vi "WVDIAL_1_AMCS_2.0.vi"() -> ()   [LabVIEW 2012]
uses:
  <vilib>/Analysis/baseanly.llb/Mean (DBL).vi
  NCAR_DIAL_Labview/AMCS_Data.vi
  AmcsUsb.dll
  <vilib>/Analysis/NI_AALBase.lvlib
panel:
  out "x/y":dbl=nan
  out "Narrow Ratio":dbl(graph)=nan
  in  "Near Ch Offline mult":dbl=0.85
  out "size(s)":i32=1121
  in  "Channels":u32=4
  in  "Data Reads":i32=279
  out "Loop Count":i32=835
  in  "TC Start":i32=2 min=1 max=1894
  in  "TC Length":i32=15 min=2 max=280
  out "TC background sub over length":cluster{dbl, dbl, dbl, dbl}(graph)={0.0, 0.0, 2617.010638297873, 3738.4361702127662}
  out "return type":i32
  out "Raw Uncorrected Return":u16[][](graph)=[[0, 0, 0, 0, 0, 0, 0, 0, 0, 0, 0, 0, 0, 0, 0, 0, 0, 0, 0, 0, 0, 0, 0, 0, 0, 0, 0, 0, 0, 0, 0, 0, 0, 0, 0, 0, 0, 0, 0, 0, 0, 0, 0, 0, 0, 0, 0, 0, 0, 0, 0, 0, 0, 0, 0, 0, 0, 0, 0, 0, 0, 0, 0, 0, 0, 0, 0, 0, 0, 0, 0, 0, 0, 0, 0, 0, 0, 0, 0, 0, 0, 0, 0, 0, 0, 0, 0, 0, 0, 0, 0, 0, 0, 0, 0, 0, 0, 0, 0, 0, 0, 0, 0, 0, 0, 0, 0, 0, 0, 0, 0, 0, 0, 0, 0, 0, 0, 0, 0, 0, 0, 0, 0, 0, 0, 0, 0, 0, 0, 0, 0, 0, 0, 0, 0, 0, 0, 0, 0, 0, 0, 0, 0, 0, 0, 0, 0, 0, 0, 0, 0, 0, 0, 0, 0, 0, 0, 0, 0, 0, 0, 0, 0, 0, 0, 0, 0, 0, 0, 0, 0, 0, 0, 0, 0, 0, 0, 0, 0, 0, 0, 0, 0, 0, 0, 0, 0, 0, 0, 0, 0, 0, 0, 0, 0, 0, 0, 0, 0, 0, 0, 0, 0, 0, 0, 0, 0, 0, 0, 0, 0, 0, 0, 0, 0, 0, 0, 0, 0, 0, 0, 0, 0, 0, 0, 0, 0, 0, 0, 0, 0, 0, 0, 0, 0, 0, 0, 0, 0, 0, 0, 0, 0, 0, 0, 0, 0, 0, 0, 0, 0, 0, 0, 0, 0, 0, 0, 0, 0, 0, 0, 0, 0, 0, 0, 0, 0, 0, 0, 0, 0, 0, 0, 0, 0, 0, 0, 0, 0, 0], [0, 0, 0, 0, 0, 0, 0, 0, 0, 0, 0, 0, 0, 0, 0, 0, 0, 0, 0, 0, 0, 0, 0, 0, 0, 0, 0, 0, 0, 0, 0, 0, 0, 0, 0, 0, 0, 0, 0, 0, 0, 0, 0, 0, 0, 0, 0, 0, 0, 0, 0, 0, 0, 0, 0, 0, 0, 0, 0, 0, 0, 0, 0, 0, 0, 0, 0, 0, 0, 0, 0, 0, 0, 0, 0, 0, 0, 0, 0, 0, 0, 0, 0, 0, 0, 0, 0, 0, 0, 0, 0, 0, 0, 0, 0, 0, 0, 0, 0, 0, 0, 0, 0, 0, 0, 0, 0, 0, 0, 0, 0, 0, 0, 0, 0, 0, 0, 0, 0, 0, 0, 0, 0, 0, 0, 0, 0, 0, 0, 0, 0, 0, 0, 0, 0, 0, 0, 0, 0, 0, 0, 0, 0, 0, 0, 0, 0, 0, 0, 0, 0, 0, 0, 0, 0, 0, 0, 0, 0, 0, 0, 0, 0, 0, 0, 0, 0, 0, 0, 0, 0, 0, 0, 0, 0, 0, 0, 0, 0, 0, 0, 0, 0, 0, 0, 0, 0, 0, 0, 0, 0, 0, 0, 0, 0, 0, 0, 0, 0, 0, 0, 0, 0, 0, 0, 0, 0, 0, 0, 0, 0, 0, 0, 0, 0, 0, 0, 0, 0, 0, 0, 0, 0, 0, 0, 0, 0, 0, 0, 0, 0, 0, 0, 0, 0, 0, 0, 0, 0, 0, 0, 0, 0, 0, 0, 0, 0, 0, 0, 0, 0, 0, 0, 0, 0, 0, 0, 0, 0, 0, 0, 0, 0, 0, 0, 0, 0, 0, 0, 0, 0, 0, 0, 0, 0, 0, 0, 0, 0, 0], [16853, 241, 204, 203, 228, 261, 282, 296, 297, 331, 349, 362, 433, 449, 460, 491, 495, 520, 510, 556, 556, 565, 611, 567, 552, 601, 573, 553, 503, 557, 470, 499, 463, 501, 449, 442, 440, 432, 426, 403, 428, 394, 399, 368, 342, 336, 322, 360, 339, 308, 315, 291, 290, 338, 318, 292, 270, 306, 296, 359, 323, 305, 218, 355, 329, 334, 295, 287, 310, 245, 230, 237, 224, 206, 277, 204, 214, 197, 167, 177, 176, 175, 173, 184, 163, 164, 174, 180, 196, 147, 167, 181, 193, 208, 206, 150, 185, 167, 150, 178, 172, 182, 165, 183, 161, 162, 174, 181, 200, 180, 169, 177, 162, 179, 185, 172, 169, 159, 172, 166, 170, 174, 163, 163, 160, 163, 189, 204, 160, 174, 158, 157, 164, 169, 180, 179, 151, 173, 160, 154, 168, 155, 177, 162, 188, 163, 177, 169, 196, 168, 156, 176, 160, 172, 156, 163, 192, 167, 173, 167, 184, 205, 179, 157, 166, 164, 152, 142, 156, 160, 167, 158, 166, 195, 171, 167, 174, 167, 185, 185, 176, 156, 172, 160, 170, 182, 183, 173, 175, 166, 192, 154, 173, 187, 154, 159, 172, 154, 159, 155, 171, 146, 162, 146, 172, 168, 179, 191, 178, 155, 160, 167, 168, 173, 165, 171, 160, 140, 199, 162, 161, 156, 176, 173, 175, 157, 167, 186, 155, 181, 171, 170, 177, 158, 194, 187, 140, 187, 150, 165, 176, 174, 178, 160, 146, 175, 149, 161, 139, 151, 168, 178, 158, 152, 185, 158, 168, 167, 190, 178, 182, 163, 189, 160, 163, 151, 186, 157, 162, 190, 168, 159, 192, 172, 163, 171, 189, 173, 158, 183], [38037, 236, 178, 171, 179, 186, 201, 209, 261, 328, 315, 386, 406, 494, 521, 567, 610, 682, 689, 654, 690, 641, 695, 703, 756, 778, 687, 701, 681, 649, 640, 585, 602, 541, 571, 498, 518, 534, 470, 446, 415, 431, 423, 351, 381, 363, 349, 345, 357, 315, 283, 311, 319, 299, 301, 253, 310, 1200, 3260, 6470, 6733, 4551, 2689, 5021, 10754, 11587, 7963, 7107, 7726, 6654, 4433, 3014, 2917, 2990, 4569, 4723, 2702, 1231, 763, 240, 130, 110, 115, 114, 97, 95, 107, 128, 212, 314, 405, 559, 837, 1180, 1188, 1033, 601, 324, 303, 501, 516, 299, 202, 141, 158, 302, 512, 633, 776, 696, 430, 239, 131, 101, 90, 80, 98, 89, 77, 76, 75, 93, 80, 95, 88, 106, 82, 99, 90, 86, 100, 87, 83, 76, 96, 87, 95, 118, 89, 77, 96, 86, 89, 92, 80, 94, 77, 91, 83, 93, 96, 85, 80, 79, 87, 91, 107, 79, 77, 84, 84, 85, 86, 84, 90, 98, 86, 97, 82, 84, 82, 73, 93, 82, 79, 79, 86, 92, 96, 97, 92, 88, 90, 76, 98, 87, 79, 79, 79, 88, 66, 93, 94, 79, 80, 83, 83, 78, 78, 75, 102, 92, 86, 89, 61, 83, 92, 87, 90, 70, 76, 78, 104, 74, 86, 86, 92, 74, 104, 103, 59, 72, 97, 86, 86, 90, 75, 93, 70, 101, 57, 89, 97, 80, 84, 89, 84, 80, 95, 90, 87, 79, 87, 82, 91, 82, 83, 79, 81, 92, 80, 81, 87, 92, 92, 82, 89, 82, 93, 79, 89, 90, 83, 87, 80, 84, 80, 116, 87, 93, 86, 79, 79, 106, 86, 90, 85, 79, 74, 91]]
  in  "stop":bool
  out "Corrected Return":dbl[][](graph)=[[0.0, 0.0, 0.0, 0.0, 0.0, 0.0, 0.0, 0.0, 0.0, 0.0, 0.0, 0.0, 0.0, 0.0, 0.0, 0.0, 0.0, 0.0, 0.0, 0.0, 0.0, 0.0, 0.0, 0.0, 0.0, 0.0, 0.0, 0.0, 0.0, 0.0, 0.0, 0.0, 0.0, 0.0, 0.0, 0.0, 0.0, 0.0, 0.0, 0.0, 0.0, 0.0, 0.0, 0.0, 0.0, 0.0, 0.0, 0.0, 0.0, 0.0, 0.0, 0.0, 0.0, 0.0, 0.0, 0.0, 0.0, 0.0, 0.0, 0.0, 0.0, 0.0, 0.0, 0.0, 0.0, 0.0, 0.0, 0.0, 0.0, 0.0, 0.0, 0.0, 0.0, 0.0, 0.0, 0.0, 0.0, 0.0, 0.0, 0.0, 0.0, 0.0, 0.0, 0.0, 0.0, 0.0, 0.0, 0.0, 0.0, 0.0, 0.0, 0.0, 0.0, 0.0, 0.0, 0.0, 0.0, 0.0, 0.0, 0.0, 0.0, 0.0, 0.0, 0.0, 0.0, 0.0, 0.0, 0.0, 0.0, 0.0, 0.0, 0.0, 0.0, 0.0, 0.0, 0.0, 0.0, 0.0, 0.0, 0.0, 0.0, 0.0, 0.0, 0.0, 0.0, 0.0, 0.0, 0.0, 0.0, 0.0, 0.0, 0.0, 0.0, 0.0, 0.0, 0.0, 0.0, 0.0, 0.0, 0.0, 0.0, 0.0, 0.0, 0.0, 0.0, 0.0, 0.0, 0.0, 0.0, 0.0, 0.0, 0.0, 0.0, 0.0, 0.0, 0.0, 0.0, 0.0, 0.0, 0.0, 0.0, 0.0, 0.0, 0.0, 0.0, 0.0, 0.0, 0.0, 0.0, 0.0, 0.0, 0.0, 0.0, 0.0, 0.0, 0.0, 0.0, 0.0, 0.0, 0.0, 0.0, 0.0, 0.0, 0.0, 0.0, 0.0, 0.0, 0.0, 0.0, 0.0, 0.0, 0.0, 0.0, 0.0, 0.0, 0.0, 0.0, 0.0, 0.0, 0.0, 0.0, 0.0, 0.0, 0.0, 0.0, 0.0, 0.0, 0.0, 0.0, 0.0, 0.0, 0.0, 0.0, 0.0, 0.0, 0.0, 0.0, 0.0, 0.0, 0.0, 0.0, 0.0, 0.0, 0.0, 0.0, 0.0, 0.0, 0.0, 0.0, 0.0, 0.0, 0.0, 0.0, 0.0, 0.0, 0.0, 0.0, 0.0, 0.0, 0.0, 0.0, 0.0, 0.0, 0.0, 0.0, 0.0, 0.0, 0.0, 0.0, 0.0, 0.0, 0.0, 0.0, 0.0, 0.0, 0.0, 0.0, 0.0, 0.0, 0.0, 0.0, 0.0, 0.0, 0.0, 0.0, 0.0, 0.0, 0.0, 0.0, 0.0, 0.0, 0.0, 0.0, 0.0, 0.0, 0.0, 0.0, 0.0, 0.0, 0.0], [0.0, 0.0, 0.0, 0.0, 0.0, 0.0, 0.0, 0.0, 0.0, 0.0, 0.0, 0.0, 0.0, 0.0, 0.0, 0.0, 0.0, 0.0, 0.0, 0.0, 0.0, 0.0, 0.0, 0.0, 0.0, 0.0, 0.0, 0.0, 0.0, 0.0, 0.0, 0.0, 0.0, 0.0, 0.0, 0.0, 0.0, 0.0, 0.0, 0.0, 0.0, 0.0, 0.0, 0.0, 0.0, 0.0, 0.0, 0.0, 0.0, 0.0, 0.0, 0.0, 0.0, 0.0, 0.0, 0.0, 0.0, 0.0, 0.0, 0.0, 0.0, 0.0, 0.0, 0.0, 0.0, 0.0, 0.0, 0.0, 0.0, 0.0, 0.0, 0.0, 0.0, 0.0, 0.0, 0.0, 0.0, 0.0, 0.0, 0.0, 0.0, 0.0, 0.0, 0.0, 0.0, 0.0, 0.0, 0.0, 0.0, 0.0, 0.0, 0.0, 0.0, 0.0, 0.0, 0.0, 0.0, 0.0, 0.0, 0.0, 0.0, 0.0, 0.0, 0.0, 0.0, 0.0, 0.0, 0.0, 0.0, 0.0, 0.0, 0.0, 0.0, 0.0, 0.0, 0.0, 0.0, 0.0, 0.0, 0.0, 0.0, 0.0, 0.0, 0.0, 0.0, 0.0, 0.0, 0.0, 0.0, 0.0, 0.0, 0.0, 0.0, 0.0, 0.0, 0.0, 0.0, 0.0, 0.0, 0.0, 0.0, 0.0, 0.0, 0.0, 0.0, 0.0, 0.0, 0.0, 0.0, 0.0, 0.0, 0.0, 0.0, 0.0, 0.0, 0.0, 0.0, 0.0, 0.0, 0.0, 0.0, 0.0, 0.0, 0.0, 0.0, 0.0, 0.0, 0.0, 0.0, 0.0, 0.0, 0.0, 0.0, 0.0, 0.0, 0.0, 0.0, 0.0, 0.0, 0.0, 0.0, 0.0, 0.0, 0.0, 0.0, 0.0, 0.0, 0.0, 0.0, 0.0, 0.0, 0.0, 0.0, 0.0, 0.0, 0.0, 0.0, 0.0, 0.0, 0.0, 0.0, 0.0, 0.0, 0.0, 0.0, 0.0, 0.0, 0.0, 0.0, 0.0, 0.0, 0.0, 0.0, 0.0, 0.0, 0.0, 0.0, 0.0, 0.0, 0.0, 0.0, 0.0, 0.0, 0.0, 0.0, 0.0, 0.0, 0.0, 0.0, 0.0, 0.0, 0.0, 0.0, 0.0, 0.0, 0.0, 0.0, 0.0, 0.0, 0.0, 0.0, 0.0, 0.0, 0.0, 0.0, 0.0, 0.0, 0.0, 0.0, 0.0, 0.0, 0.0, 0.0, 0.0, 0.0, 0.0, 0.0, 0.0, 0.0, 0.0, 0.0, 0.0, 0.0, 0.0, 0.0, 0.0, 0.0, 0.0, 0.0, 0.0, 0.0, 0.0, 0.0, 0.0, 0.0, 0.0, 0.0, 0.0, 0.0, 0.0], [16684.73404255319, 72.7340425531915, 35.7340425531915, 34.7340425531915, 59.7340425531915, 92.7340425531915, 113.7340425531915, 127.7340425531915, 128.7340425531915, 162.7340425531915, 180.7340425531915, 193.7340425531915, 264.7340425531915, 280.7340425531915, 291.7340425531915, 322.7340425531915, 326.7340425531915, 351.7340425531915, 341.7340425531915, 387.7340425531915, 387.7340425531915, 396.7340425531915, 442.7340425531915, 398.7340425531915, 383.7340425531915, 432.7340425531915, 404.7340425531915, 384.7340425531915, 334.7340425531915, 388.7340425531915, 301.7340425531915, 330.7340425531915, 294.7340425531915, 332.7340425531915, 280.7340425531915, 273.7340425531915, 271.7340425531915, 263.7340425531915, 257.7340425531915, 234.7340425531915, 259.7340425531915, 225.7340425531915, 230.7340425531915, 199.7340425531915, 173.7340425531915, 167.7340425531915, 153.7340425531915, 191.7340425531915, 170.7340425531915, 139.7340425531915, 146.7340425531915, 122.7340425531915, 121.7340425531915, 169.7340425531915, 149.7340425531915, 123.7340425531915, 101.7340425531915, 137.7340425531915, 127.7340425531915, 190.7340425531915, 154.7340425531915, 136.7340425531915, 49.7340425531915, 186.7340425531915, 160.7340425531915, 165.7340425531915, 126.7340425531915, 118.7340425531915, 141.7340425531915, 76.7340425531915, 61.7340425531915, 68.7340425531915, 55.7340425531915, 37.7340425531915, 108.7340425531915, 35.7340425531915, 45.7340425531915, 28.7340425531915, -1.2659574468084998, 8.7340425531915, 7.7340425531915, 6.7340425531915, 4.7340425531915, 15.7340425531915, -5.2659574468085, -4.2659574468085, 5.7340425531915, 11.7340425531915, 27.7340425531915, -21.2659574468085, -1.2659574468084998, 12.7340425531915, 24.7340425531915, 39.7340425531915, 37.7340425531915, -18.2659574468085, 16.7340425531915, -1.2659574468084998, -18.2659574468085, 9.7340425531915, 3.7340425531915002, 13.7340425531915, -3.2659574468084998, 14.7340425531915, -7.2659574468085, -6.2659574468085, 5.7340425531915, 12.7340425531915, 31.7340425531915, 11.7340425531915, 0.7340425531915002, 8.7340425531915, -6.2659574468085, 10.7340425531915, 16.7340425531915, 3.7340425531915002, 0.7340425531915002, -9.2659574468085, 3.7340425531915002, -2.2659574468084998, 1.7340425531915002, 5.7340425531915, -5.2659574468085, -5.2659574468085, -8.2659574468085, -5.2659574468085, 20.7340425531915, 35.7340425531915, -8.2659574468085, 5.7340425531915, -10.2659574468085, -11.2659574468085, -4.2659574468085, 0.7340425531915002, 11.7340425531915, 10.7340425531915, -17.2659574468085, 4.7340425531915, -8.2659574468085, -14.2659574468085, -0.26595744680849975, -13.2659574468085, 8.7340425531915, -6.2659574468085, 19.7340425531915, -5.2659574468085, 8.7340425531915, 0.7340425531915002, 27.7340425531915, -0.26595744680849975, -12.2659574468085, 7.7340425531915, -8.2659574468085, 3.7340425531915002, -12.2659574468085, -5.2659574468085, 23.7340425531915, -1.2659574468084998, 4.7340425531915, -1.2659574468084998, 15.7340425531915, 36.7340425531915, 10.7340425531915, -11.2659574468085, -2.2659574468084998, -4.2659574468085, -16.2659574468085, -26.2659574468085, -12.2659574468085, -8.2659574468085, -1.2659574468084998, -10.2659574468085, -2.2659574468084998, 26.7340425531915, 2.7340425531915002, -1.2659574468084998, 5.7340425531915, -1.2659574468084998, 16.7340425531915, 16.7340425531915, 7.7340425531915, -12.2659574468085, 3.7340425531915002, -8.2659574468085, 1.7340425531915002, 13.7340425531915, 14.7340425531915, 4.7340425531915, 6.7340425531915, -2.2659574468084998, 23.7340425531915, -14.2659574468085, 4.7340425531915, 18.7340425531915, -14.2659574468085, -9.2659574468085, 3.7340425531915002, -14.2659574468085, -9.2659574468085, -13.2659574468085, 2.7340425531915002, -22.2659574468085, -6.2659574468085, -22.2659574468085, 3.7340425531915002, -0.26595744680849975, 10.7340425531915, 22.7340425531915, 9.7340425531915, -13.2659574468085, -8.2659574468085, -1.2659574468084998, -0.26595744680849975, 4.7340425531915, -3.2659574468084998, 2.7340425531915002, -8.2659574468085, -28.2659574468085, 30.7340425531915, -6.2659574468085, -7.2659574468085, -12.2659574468085, 7.7340425531915, 4.7340425531915, 6.7340425531915, -11.2659574468085, -1.2659574468084998, 17.7340425531915, -13.2659574468085, 12.7340425531915, 2.7340425531915002, 1.7340425531915002, 8.7340425531915, -10.2659574468085, 25.7340425531915, 18.7340425531915, -28.2659574468085, 18.7340425531915, -18.2659574468085, -3.2659574468084998, 7.7340425531915, 5.7340425531915, 9.7340425531915, -8.2659574468085, -22.2659574468085, 6.7340425531915, -19.2659574468085, -7.2659574468085, -29.2659574468085, -17.2659574468085, -0.26595744680849975, 9.7340425531915, -10.2659574468085, -16.2659574468085, 16.7340425531915, -10.2659574468085, -0.26595744680849975, -1.2659574468084998, 21.7340425531915, 9.7340425531915, 13.7340425531915, -5.2659574468085, 20.7340425531915, -8.2659574468085, -5.2659574468085, -17.2659574468085, 17.7340425531915, -11.2659574468085, -6.2659574468085, 21.7340425531915, -0.26595744680849975, -9.2659574468085, 23.7340425531915, 3.7340425531915002, -5.2659574468085, 2.7340425531915002, 20.7340425531915, 4.7340425531915, -10.2659574468085, 14.7340425531915], [32259.281382978723, 128.4313829787234, 79.13138297872341, 73.1813829787234, 79.9813829787234, 85.9313829787234, 98.6813829787234, 105.4813829787234, 149.6813829787234, 206.6313829787234, 195.58138297872338, 255.93138297872338, 272.9313829787234, 347.7313829787234, 370.6813829787234, 409.7813829787234, 446.3313829787234, 507.53138297872346, 513.4813829787234, 483.73138297872345, 514.3313829787235, 472.68138297872343, 518.5813829787235, 525.3813829787234, 570.4313829787234, 589.1313829787234, 511.78138297872346, 523.6813829787234, 506.68138297872343, 479.48138297872345, 471.8313829787234, 425.0813829787234, 439.53138297872346, 387.6813829787234, 413.1813829787234, 351.13138297872337, 368.13138297872337, 381.7313829787234, 327.3313829787234, 306.9313829787234, 280.5813829787234, 294.1813829787234, 287.38138297872337, 226.18138297872338, 251.68138297872338, 236.3813829787234, 224.4813829787234, 221.08138297872338, 231.2813829787234, 195.58138297872338, 168.3813829787234, 192.1813829787234, 198.9813829787234, 181.9813829787234, 183.6813829787234, 142.8813829787234, 191.33138297872338, 947.8313829787235, 2698.8313829787235, 5427.331382978723, 5650.881382978723, 3796.181382978723, 2213.4813829787236, 4195.681382978723, 9068.731382978724, 9776.781382978723, 6696.381382978723, 5968.781382978723, 6494.9313829787225, 5583.731382978723, 3695.8813829787227, 2489.7313829787236, 2407.2813829787233, 2469.3313829787235, 3811.481382978723, 3942.3813829787227, 2224.5313829787233, 974.1813829787234, 576.3813829787234, 131.83138297872338, 38.33138297872341, 21.331382978723408, 25.581382978723408, 24.73138297872341, 10.281382978723409, 8.58138297872341, 18.781382978723407, 36.63138297872341, 108.0313829787234, 194.7313829787234, 272.0813829787234, 402.9813829787234, 639.2813829787234, 930.8313829787235, 937.6313829787234, 805.8813829787234, 438.68138297872343, 203.2313829787234, 185.3813829787234, 353.6813829787234, 366.4313829787234, 181.9813829787234, 99.5313829787234, 47.681382978723406, 62.13138297872341, 184.5313829787234, 363.0313829787234, 465.8813829787234, 587.4313829787234, 519.4313829787234, 293.3313829787234, 130.9813829787234, 39.181382978723406, 13.68138297872341, 4.331382978723409, -4.1686170212765905, 11.131382978723408, 3.481382978723409, -6.71861702127659, -7.568617021276591, -8.41861702127659, 6.881382978723409, -4.1686170212765905, 8.58138297872341, 2.631382978723409, 17.93138297872341, -2.4686170212765908, 11.981382978723408, 4.331382978723409, 0.9313829787234091, 12.83138297872341, 1.781382978723409, -1.618617021276591, -7.568617021276591, 9.43138297872341, 1.781382978723409, 8.58138297872341, 28.13138297872341, 3.481382978723409, -6.71861702127659, 9.43138297872341, 0.9313829787234091, 3.481382978723409, 6.031382978723409, -4.1686170212765905, 7.731382978723409, -6.71861702127659, 5.181382978723409, -1.618617021276591, 6.881382978723409, 9.43138297872341, 0.08138297872340913, -4.1686170212765905, -5.018617021276591, 1.781382978723409, 5.181382978723409, 18.781382978723407, -5.018617021276591, -6.71861702127659, -0.7686170212765908, -0.7686170212765908, 0.08138297872340913, 0.9313829787234091, -0.7686170212765908, 4.331382978723409, 11.131382978723408, 0.9313829787234091, 10.281382978723409, -2.4686170212765908, -0.7686170212765908, -2.4686170212765908, -10.11861702127659, 6.881382978723409, -2.4686170212765908, -5.018617021276591, -5.018617021276591, 0.9313829787234091, 6.031382978723409, 9.43138297872341, 10.281382978723409, 6.031382978723409, 2.631382978723409, 4.331382978723409, -7.568617021276591, 11.131382978723408, 1.781382978723409, -5.018617021276591, -5.018617021276591, -5.018617021276591, 2.631382978723409, -16.06861702127659, 6.881382978723409, 7.731382978723409, -5.018617021276591, -4.1686170212765905, -1.618617021276591, -1.618617021276591, -5.868617021276591, -5.868617021276591, -8.41861702127659, 14.531382978723409, 6.031382978723409, 0.9313829787234091, 3.481382978723409, -20.31861702127659, -1.618617021276591, 6.031382978723409, 1.781382978723409, 4.331382978723409, -12.66861702127659, -7.568617021276591, -5.868617021276591, 16.23138297872341, -9.26861702127659, 0.9313829787234091, 0.9313829787234091, 6.031382978723409, -9.26861702127659, 16.23138297872341, 15.381382978723408, -22.01861702127659, -10.968617021276591, 10.281382978723409, 0.9313829787234091, 0.9313829787234091, 4.331382978723409, -8.41861702127659, 6.881382978723409, -12.66861702127659, 13.68138297872341, -23.71861702127659, 3.481382978723409, 10.281382978723409, -4.1686170212765905, -0.7686170212765908, 3.481382978723409, -0.7686170212765908, -4.1686170212765905, 8.58138297872341, 4.331382978723409, 1.781382978723409, -5.018617021276591, 1.781382978723409, -2.4686170212765908, 5.181382978723409, -2.4686170212765908, -1.618617021276591, -5.018617021276591, -3.318617021276591, 6.031382978723409, -4.1686170212765905, -3.318617021276591, 1.781382978723409, 6.031382978723409, 6.031382978723409, -2.4686170212765908, 3.481382978723409, -2.4686170212765908, 6.881382978723409, -5.018617021276591, 3.481382978723409, 4.331382978723409, -1.618617021276591, 1.781382978723409, -4.1686170212765905, -0.7686170212765908, -4.1686170212765905, 26.43138297872341, 1.781382978723409, 6.881382978723409, 0.9313829787234091, -5.018617021276591, -5.018617021276591, 17.93138297872341, 0.9313829787234091, 4.331382978723409, 0.08138297872340913, -5.018617021276591, -9.26861702127659, 5.181382978723409]] caption="Corrected Signal"
  out "Max. Rep. Rate (Hz)":dbl=7091.695624423801
  out "Data Collection Time per Column":dbl=2.00004285
  out "Minimum Sync Pulse Period(µs)":dbl=141.01 format="%.2f"
  in  "y units":u16(ring) items=["Bin #", "Sampling Time(µs)", "Range(m)"]
  in  "Time Resolution Per Bin(ns)":u16=500 min=5 max=1063 step=1
  in  "Number of Accumulates":u32=14285 min=1 max=32767 step=1
  in  "Pulse A Polarity":enum16{"Low", "High"}(ring)=enum."High"
  in  "Sync Pulse Polarity":enum32{"Low", "High"}(ring)=enum."High"
  in  "Accumulation Delay(ns)":u16=10 min=10 max=1270 step=1
  in  "Pulse B Delay(ns)":u32=170000 min=80 max=327600 step=1
  in  "Pulse A Delay(ns)":u32=1040 min=80 max=327600
  in  "bins":u32=280 min=2 max=4095 step=1
  out "y offset":u16=10
  in  "ns scale":u16=500
  in  "Pulse B Polarity":enum16{"Low", "High"}(ring)=enum."High"
  out "Running?":bool
  out "Device ID":u32
  out "Open?":bool=TRUE
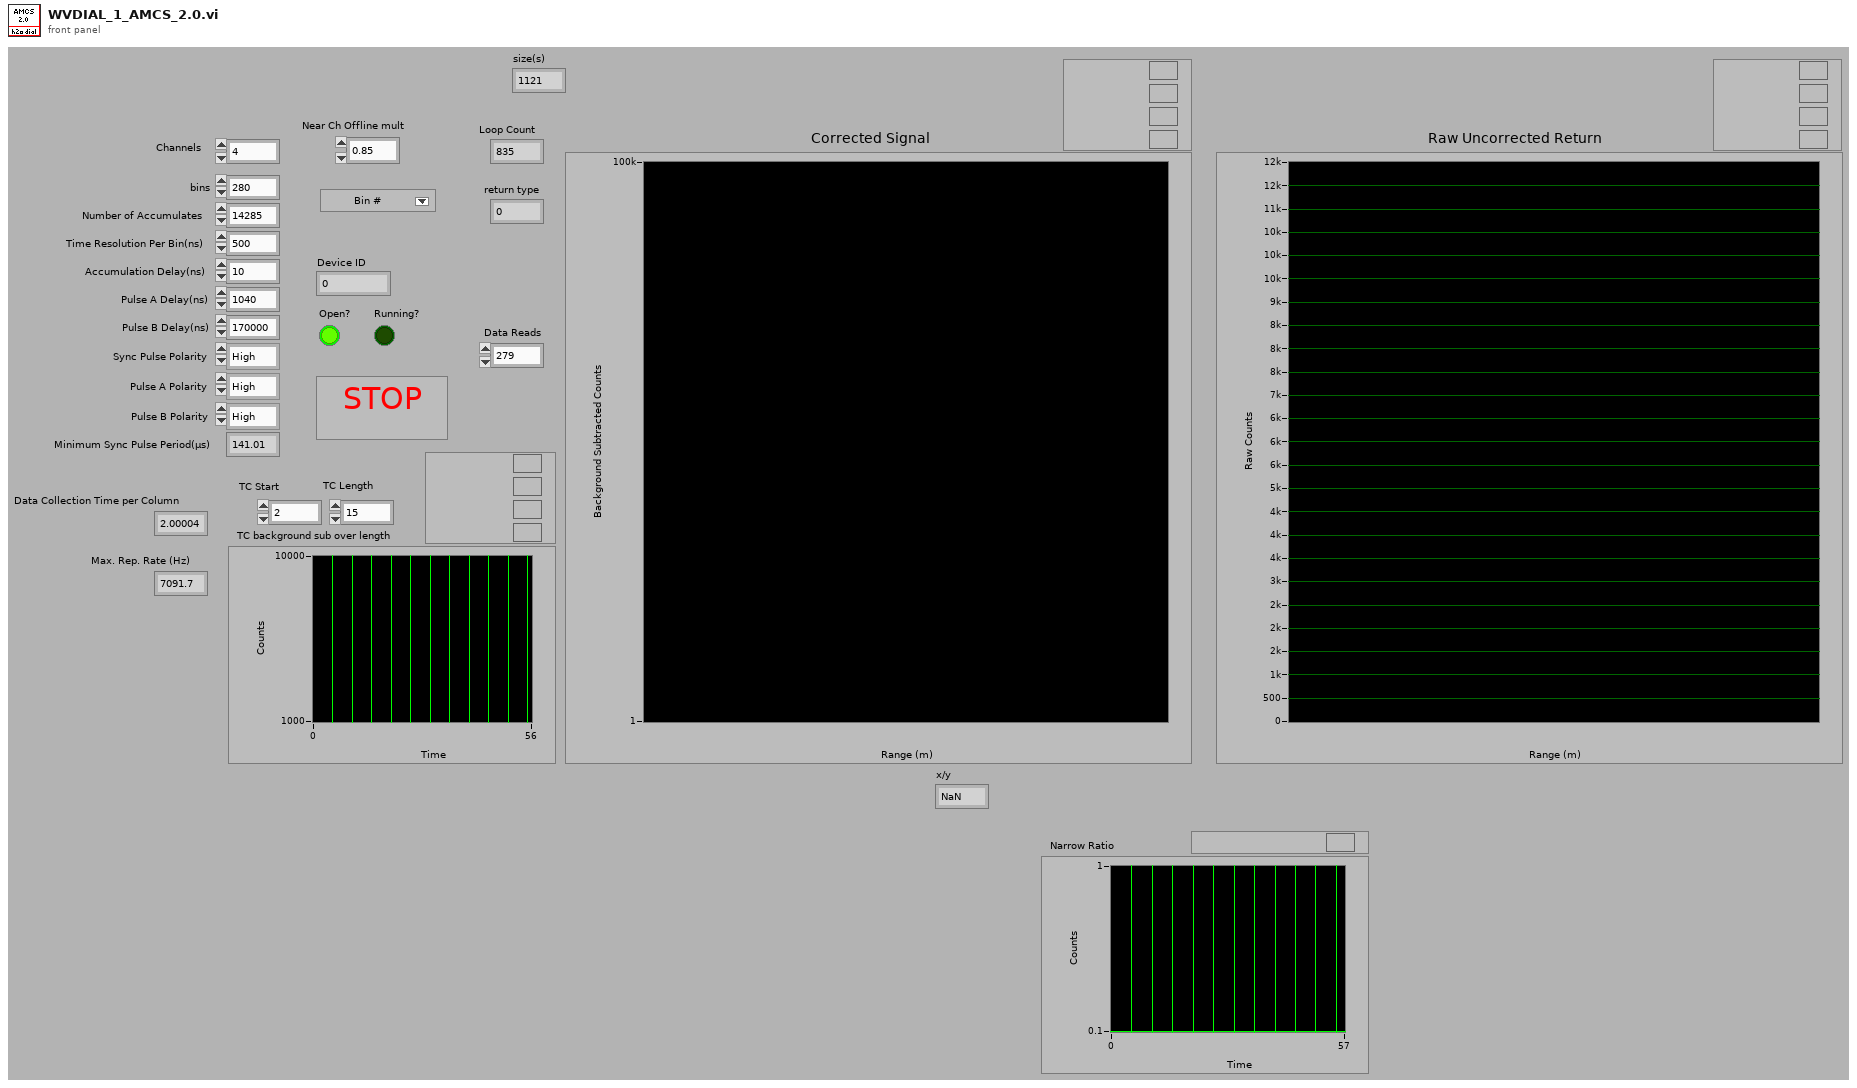
[diagram p1: front panel]
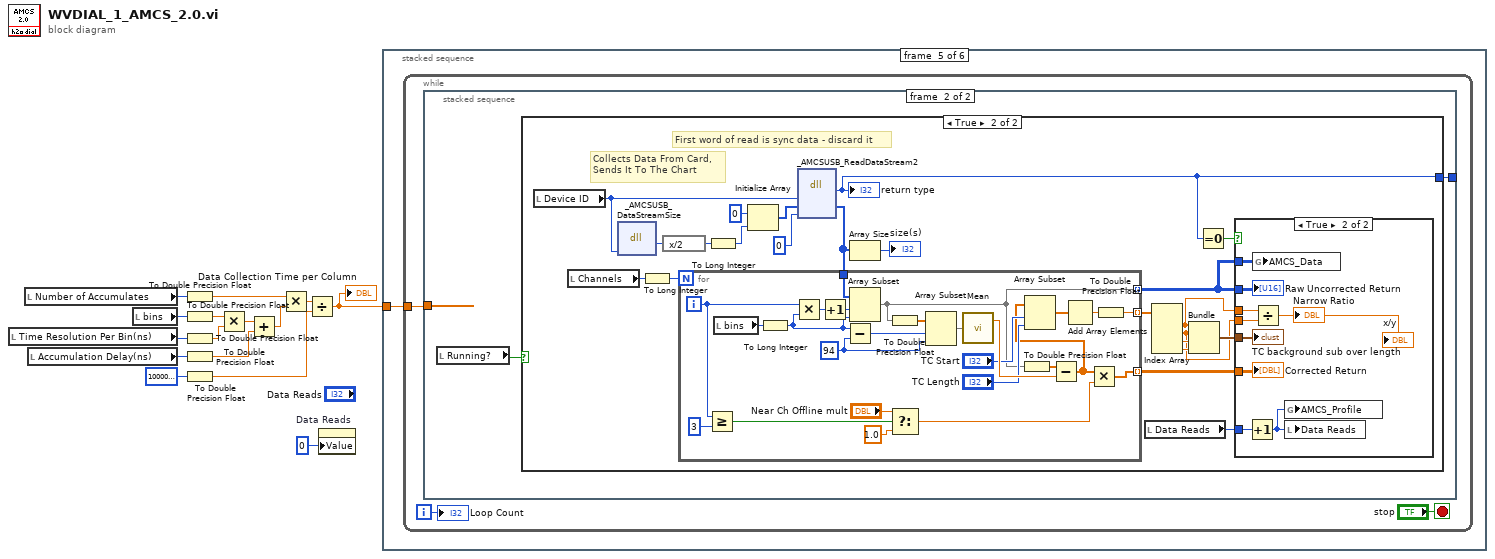
[diagram p0: block diagram]
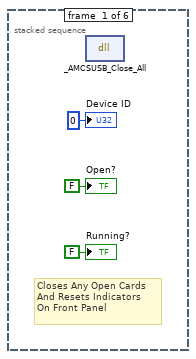
[diagram p2: hidden frame]
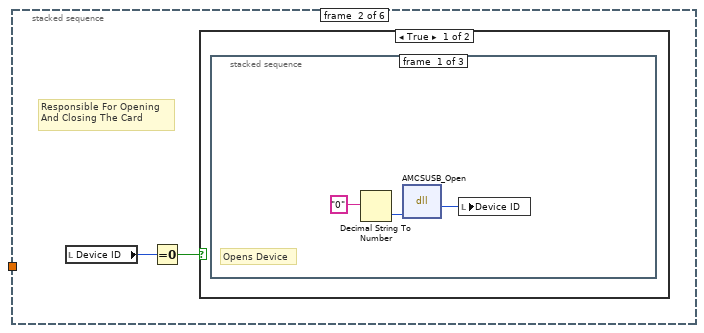
[diagram p3: hidden frame]
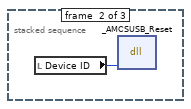
[diagram p4: hidden frame]
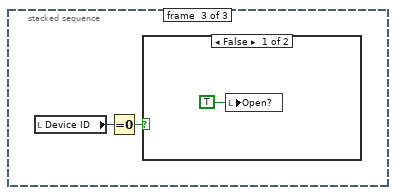
[diagram p5: hidden frame]
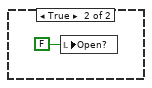
[diagram p6: hidden frame]
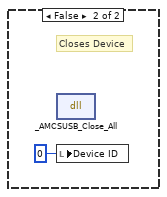
[diagram p7: hidden frame]
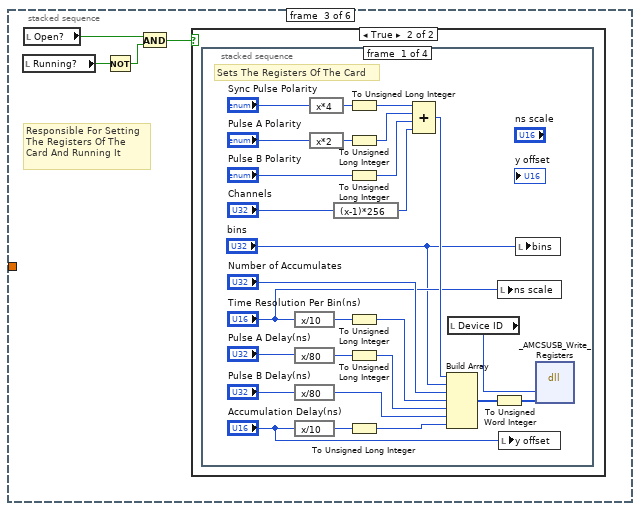
[diagram p8: hidden frame]
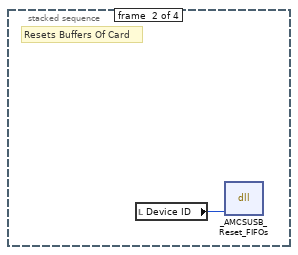
[diagram p10: hidden frame]
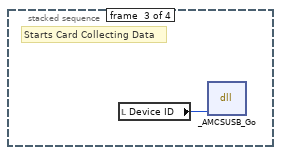
[diagram p11: hidden frame]
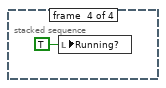
[diagram p12: hidden frame]
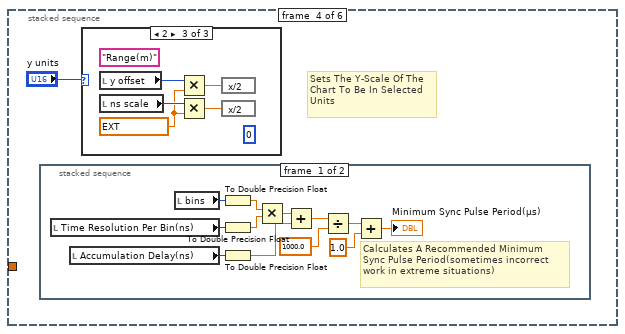
[diagram p13: hidden frame]
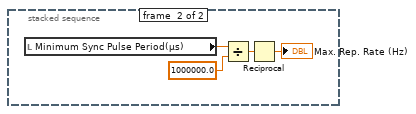
[diagram p14: hidden frame]
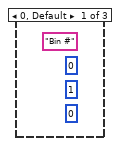
[diagram p15: hidden frame]
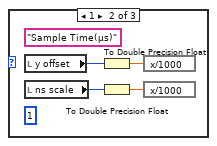
[diagram p16: hidden frame]
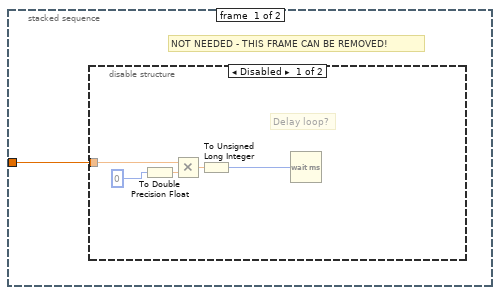
[diagram p17: hidden frame]
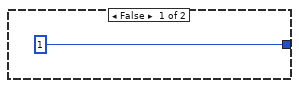
[diagram p19: hidden frame]
diagram:
  n1 = local read "Time Resolution Per Bin(ns)"() -> (w4:u16)
  n2 = local read "Number of Accumulates"() -> (w11:u32)
  n3 = local read "Accumulation Delay(ns)"() -> (w2:u16)
  n4 = local read "bins"() -> (w6:u32)
  n5 = To Double Precision Float(number=w11) -> (double precision float=w10:dbl)
  n6 = To Double Precision Float(number=w6) -> (double precision float=w5:dbl)
  n7 = To Double Precision Float(number=w4) -> (double precision float=w7:dbl)
  n8 = To Double Precision Float(number=w2) -> (double precision float=w3:dbl)
  n9 = To Double Precision Float(number=1000000000) -> (double precision float=w8:dbl)
  n10 = Multiply(x=w5, y=w7) -> (x*y=w15:dbl)
  n11 = Add(x=w15, y=w3) -> (x+y=w14:dbl)
  n12 = Multiply(x=w10, y=w14) -> (x*y=w13:dbl)
  n13 = Divide(x=w13, y=w8) -> (x/y=w12:dbl)
  "Data Collection Time per Column" <- w12
  n14 = property on="Data Reads" class="DigNum (strict)"("Value"=0 ("Data Reads")) -> ()  [unwired: 2 in, 2 out]
  n15 = stacked-sequence {
    tunnel: w12 -> [_ _ _ _ w90 _]
    frame #0 {
      # "Closes Any Open Cards\nAnd Resets Indicators\nOn Front Panel"
      n16 = dll-call lib="AmcsUsb.dll" fn="_AMCSUSB_Close_All" label="Close_All"() -> ()  [unwired: 4 in, 2 out]
      "Open?" <- FALSE ("Open?")
      "Device ID" <- u32 0 ("Device ID")
      "Running?" <- FALSE ("Running?")
    }
    frame #1 {
      # "Responsible For Opening\nAnd Closing The Card"
      n17 = local read "Device ID"() -> (w20:u32)
      n18 = Equal To 0?(x=w20) -> (x = 0?=w19:bool)
      n19 = case shown="True" w19 {
        frame True {
          # "Opens Device"
          n20 = stacked-sequence {
            frame #0 {
              n21 = Decimal String To Number(string="0" ("Device Number")) -> (number=w21:i32)  [unwired: 2 in, 1 out]
              n22 = dll-call lib="AmcsUsb.dll" fn="AMCSUSB_Open"("devnum"=w21) -> ("return type"=w22:u32)  [unwired: 4 in, 2 out]
              n23 = local write "Device ID"(w22) -> ()
            }
            frame #1 {
              n24 = local read "Device ID"() -> (w24:u32)
              n25 = dll-call lib="AmcsUsb.dll" fn="_AMCSUSB_Reset" label="Reset"("handle"=w24) -> ()  [unwired: 5 in, 2 out]
            }
            frame #2 {
              n26 = local read "Device ID"() -> (w25:u32)
              n27 = Equal To 0?(x=w25) -> (x = 0?=w26:bool)
              n28 = case shown="False" w26 {
                frame False {
                  n29 = local write "Open?"(TRUE ("Open?")) -> ()
                }
                frame True {
                  n30 = local write "Open?"(FALSE ("Open?")) -> ()
                }
              }
            }
          }
        }
        frame False {
          # "Closes Device"
          n31 = dll-call lib="AmcsUsb.dll" fn="_AMCSUSB_Close_All" label="Close_All"() -> ()  [unwired: 4 in, 2 out]
          n32 = local write "Device ID"(u32 0 ("Device ID")) -> ()
        }
      }
    }
    frame #2 {
      # "Responsible For Setting\nThe Registers Of The\nCard And Running It"
      n33 = local read "Running?"() -> (w32:bool)
      n34 = local read "Open?"() -> (w33:bool)
      n35 = Not(x=w32) -> (.not. x?=w31:bool)
      n36 = And(x=w33, y=w31) -> (x .and. y?=w30:bool)
      n37 = case shown="True" w30 {
        frame False {
        }
        frame True {
          n38 = stacked-sequence {
            frame #0 {
              # "Sets The Registers Of The Card"
              n39 = expression code="x/10"("Time Resolution Per Bin(ns)") -> (w38:u16)
              n40 = expression code="x/80"("Pulse A Delay(ns)") -> (w40:u32)
              n41 = expression code="x/80"("Pulse B Delay(ns)") -> (w60:u32)
              n42 = expression code="x/10"("Accumulation Delay(ns)") -> (w42:u16)
              n43 = expression code="x*4"("Sync Pulse Polarity") -> (w47:enum32{"Low", "High"})
              n44 = expression code="x*2"("Pulse A Polarity") -> (w46:enum16{"Low", "High"})
              n45 = expression code="(x-1)*256"("Channels") -> (w54:u32)
              n46 = To Unsigned Long Integer(number=w47) -> (unsigned 32bit integer=w48:u32)
              n47 = To Unsigned Long Integer(number=w46) -> (unsigned 32bit integer=w45:u32)
              n48 = To Unsigned Long Integer(number="Pulse B Polarity") -> (unsigned 32bit integer=w43:u32)
              n49 = To Unsigned Long Integer(number=w38) -> (unsigned 32bit integer=w37:u32)
              n50 = To Unsigned Long Integer(number=w40) -> (unsigned 32bit integer=w39:u32)
              n51 = To Unsigned Long Integer(number=w42) -> (unsigned 32bit integer=w41:u32)
              n52 = Compound Arithmetic op=ADD(w48, w45, w43, w54) -> (w59:u32)
              n53 = Build Array(w59, "bins", "Number of Accumulates", w37, w39, w60, w41) -> (w36:u32[])
              n54 = local read "Device ID"() -> (w52:u32)
              n55 = To Unsigned Word Integer(number=w36) -> (unsigned 16bit integer=w35:u16[])
              n56 = local write "ns scale"("Time Resolution Per Bin(ns)") -> ()
              n57 = local write "y offset"("Accumulation Delay(ns)") -> ()
              n58 = local write "bins"("bins") -> ()
              n59 = dll-call lib="AmcsUsb.dll" fn="_AMCSUSB_Write_Registers" label="Write_Registers"("handle"=w52, "registers"=w35) -> ()  [unwired: 6 in, 2 out]
            }
            frame #1 {
              # "Resets Buffers Of Card"
              n60 = local read "Device ID"() -> (w61:u32)
              n61 = dll-call lib="AmcsUsb.dll" fn="_AMCSUSB_Reset_FIFOs" label="Reset_FIFOs"("handle"=w61) -> ()  [unwired: 5 in, 2 out]
            }
            frame #2 {
              # "Starts Card Collecting Data"
              n62 = local read "Device ID"() -> (w62:u32)
              n63 = dll-call lib="AmcsUsb.dll" fn="_AMCSUSB_Go" label="Go"("handle"=w62) -> ()  [unwired: 5 in, 2 out]
            }
            frame #3 {
              n64 = local write "Running?"(TRUE) -> ()
            }
          }
        }
      }
    }
    frame #3 {
      # "Sets The Y-Scale Of The\nChart To Be In Selected\nUnits"
      n65 = stacked-sequence {
        frame #0 {
          # "Calculates A Recommended Minimum\nSync Pulse Period(sometimes incorrect\nwork in extreme situations)"
          n66 = local read "Time Resolution Per Bin(ns)"() -> (w71:u16)
          n67 = local read "Accumulation Delay(ns)"() -> (w73:u16)
          n68 = local read "bins"() -> (w72:u32)
          n69 = To Double Precision Float(number=w72) -> (double precision float=w74:dbl)
          n70 = To Double Precision Float(number=w71) -> (double precision float=w75:dbl)
          n71 = To Double Precision Float(number=w73) -> (double precision float=w76:dbl)
          n72 = Multiply(x=w74, y=w75) -> (x*y=w70:dbl)
          n73 = Add(x=w70, y=w76) -> (x+y=w68:dbl)
          n74 = Divide(x=w68, y=1000.0) -> (x/y=w67:dbl)
          n75 = Add(x=w67, y=1.0) -> (x+y=→"Minimum Sync Pulse Period(µs)":dbl)
        }
        frame #1 {
          n76 = local read "Minimum Sync Pulse Period(µs)"() -> (w78:dbl)
          n77 = Divide(x=w78, y=1000000.0) -> (x/y=w77:dbl)
          n78 = Reciprocal(x=w77) -> (1/x=→"Max. Rep. Rate (Hz)":dbl)
        }
      }
      n79 = case shown="2" "y units" {
        frame 0, Default {
          (unwired) u8 0 ("Y Scale.Format & Precision:Precision")
          (unwired) u16 1 ("Y Scale.Offset and Multiplier:Multiplier")
          (unwired) "Bin #" ("Y Scale.Name Label.Text")
          (unwired) u16 0 ("Y Scale.Offset and Multiplier:Offset")
        }
        frame 1 {
          (unwired) u8 1 ("Y Scale.Format & Precision:Precision")
          (unwired) "Sample Time(µs)" ("Y Scale.Name Label.Text")
          n80 = local read "y offset"() -> (w84:u16)
          n81 = local read "ns scale"() -> (w83:u16)
          n82 = To Double Precision Float(number=w84) -> (double precision float=w82:dbl)
          n83 = To Double Precision Float(number=w83) -> (double precision float=w81:dbl)
          n84 = expression code="x/1000"(w82) -> ()  [unwired: 1 out]
          n85 = expression code="x/1000"(w81) -> ()  [unwired: 1 out]
        }
        frame 2 {
          (unwired) u8 0 ("Y Scale.Format & Precision:Precision")
          w85 = ext 0.299792458 ("y")
          (unwired) "Range(m)" ("Y Scale.Name Label.Text")
          n86 = local read "y offset"() -> (w88:u16)
          n87 = local read "ns scale"() -> (w89:u16)
          n88 = Multiply(x=w88, y=w85) -> (x*y=w87:ext)
          n89 = Multiply(x=w89, y=w85) -> (x*y=w86:ext)
          n90 = expression code="x/2"(w87) -> ()  [unwired: 1 out]
          n91 = expression code="x/2"(w86) -> ()  [unwired: 1 out]
        }
      }
    }
    frame #4 {
      n92 = while {
        tunnel: w90 -> [w93]
        i -> [w91]
        stop <- "stop" stop-if-true
        n93 = stacked-sequence {
          tunnel: w93 -> [w94 _]
          tunnel: [_ w100] -> _
          frame #0 {
            # "NOT NEEDED - THIS FRAME CAN BE REMOVED!"
            n94 = disable-structure shown="Disabled" {
              disable-tunnel: w94 -> [w99 _]
              frame Disabled {
                # "Delay loop?"
                n95 = To Double Precision Float(number=0) -> (double precision float=w97:dbl)
                n96 = Multiply(x=w99, y=w97) -> (x*y=w96:dbl)
                n97 = To Unsigned Long Integer(number=w96) -> (unsigned 32bit integer=w95:u32)
                n98 = Wait (ms)(milliseconds to wait=w95) -> ()  [unwired: 1 out]
              }
              frame Enabled {
              }
            }
          }
          frame #1 {
            n99 = local read "Running?"() -> (w101:bool)
            n100 = case shown="True" w101 {
              tunnel: [1 ("return type") w109] -> w100
              frame False {
              }
              frame True {
                # "First word of read is sync data - discard it"
                # "Collects Data From Card,\nSends It To The Chart"
                n101 = local read "Device ID"() -> (w121:u32)
                n102 = local read "Channels"() -> (w113:u32)
                n103 = dll-call lib="AmcsUsb.dll" fn="_AMCSUSB_DataStreamSize" label="DataStreamSize"("handle"=w121) -> ("return type"=w120:u16)  [unwired: 4 in, 2 out]
                n104 = To Long Integer(number=w113) -> (32bit integer=w114:i32)
                n105 = expression code="x/2"(w120) -> (w119:u16)
                n106 = To Long Integer(number=w119) -> (32bit integer=w118:i32)
                n107 = Initialize Array(u32 0 ("element"), w118) -> (w122:u32[])
                n108 = dll-call lib="AmcsUsb.dll" fn="_AMCSUSB_ReadDataStream2" label="ReadDataStream2"("handle"=w121, "buffer"=w122, "BytesReturned"=u32 0) -> ("return type"=w109:i32, "buffer"=w108:u16[])  [unwired: 5 in, 2 out]
                "return type" <- w109
                n109 = for {
                  N: w114 -> [_]
                  tunnel: [w133] -> w112 mode=indexing
                  tunnel: [w132] -> w117 mode=indexing
                  tunnel: [w135] -> w106 mode=indexing
                  tunnel: w108 -> [w139]
                  i -> [w126]
                  w141 = 94 ("y")
                  n110 = Greater Or Equal?(x=w126, y=3) -> (x >= y?=w130:bool)
                  n111 = local read "bins"() -> (w145:u32)
                  n112 = To Long Integer(number=w145) -> (32bit integer=w143:i32)
                  n113 = Multiply(x=w126, y=w143) -> (x*y=w144:i32)
                  n114 = Increment(x=w144) -> (x+1=w138:i32)
                  n115 = Subtract(x=w143, y=w141) -> (x-y=w142:i32)
                  n116 = Array Subset(array=w139, index=w138, length=w143) -> (w135:u16[])
                  n117 = To Double Precision Float(number=w135) -> (double precision float=w134:dbl[])
                  n118 = Select(t="Near Ch Offline mult", s=w130, f=1.0 ("y")) -> (s? t:f=w127:dbl)
                  n119 = Array Subset(array=w134, index=w142, length=w141) -> (w149:dbl[])
                  n120 = call-poly <vilib>:"Mean.vi"("X"=w149) -> ("mean"=w147:dbl)  [unwired: 1 out]
                  n121 = To Double Precision Float(number=w135) -> (double precision float=w146:dbl[])
                  n122 = Subtract(x=w146, y=w147) -> (x-y=w125:dbl[])
                  n123 = Array Subset(array=w125, index="TC Start", length="TC Length") -> (w148:dbl[])
                  n124 = Add Array Elements(numeric array=w148) -> (sum=w140:dbl)
                  n125 = Multiply(x=w125, y=w127) -> (x*y=w132:dbl[])
                  n126 = To Double Precision Float(number=w140) -> (double precision float=w133:dbl)
                }
                n127 = Array Size(array=w108) -> (size(s)=→"size(s)":i32)
                n128 = local read "Data Reads"() -> (w105:i32)
                n129 = Index Array(array=w112) -> (element #1=w104:dbl, element #2=w103:dbl, element #3=w111:dbl, element #4=w110:dbl)  [unwired: 4 in]
                n130 = Bundle(w104, w103, w111, w110) -> (w115:cluster{dbl, dbl, dbl, dbl})  [unwired: 1 in]
                n131 = Equal To 0?(x=w109) -> (x = 0?=w116:bool)
                n132 = case shown="True" w116 {
                  tunnel: w117 -> [_ w158]
                  tunnel: w106 -> [_ w157]
                  tunnel: w115 -> [_ w156]
                  tunnel: w106 -> [_ w155]
                  tunnel: w105 -> [_ w154]
                  tunnel: w104 -> [_ w151]
                  tunnel: w103 -> [_ w150]
                  frame False {
                  }
                  frame True {
                    n133 = Increment(x=w154) -> (x+1=w153:i32)
                    n134 = global write "AMCS_Data.vi" "AMCS_Data"(w155) -> ()
                    n135 = Divide(x=w151, y=w150) -> (x/y=→"Narrow Ratio" →"x/y":dbl)
                    n136 = global write "AMCS_Data.vi" "AMCS_Profile"(w153) -> ()
                    n137 = local write "Data Reads"(w153) -> ()
                    "Corrected Return" <- w158
                    "Raw Uncorrected Return" <- w157
                    "TC background sub over length" <- w156
                  }
                }
              }
            }
          }
        }
        "Loop Count" <- w91
      }
    }
    frame #5 {
      # "Closes Any Open Cards\nAnd Resets Indicators\nOn Front Panel"
      n138 = dll-call lib="AmcsUsb.dll" fn="_AMCSUSB_Close_All" label="Close_All"() -> ()  [unwired: 4 in, 2 out]
      n139 = local write "Device ID"(u32 0 ("Device ID")) -> ()
      n140 = local write "Open?"(TRUE ("Open?")) -> ()
      n141 = local write "Running?"(FALSE ("Running?")) -> ()
    }
  }
